vi "readRadonHtml.vi"(7 "Web(T)":bool=TRUE, 8 "Error In":errorcluster, 11 "url":string="http://localhost:80/radon.txt") -> (0 "Error Out":errorcluster, 1 "fechaMeas":string="17:44", 2 "fechaRead":string="25/05/1951", 3 "datoNuevo?":bool=TRUE, 4 "datosGraficaRadon":T1={"Radon"=0.0, "Temperature"=1100.0, "Humidity"=1050.25, "Pressure"=985.0, "Empty5"=885.75, "Empty6"=901.5, "Empty7"=970.5, "Empty8"=900.5} {"Empty8" format="%.1f"; "Empty7" format="%.1f"; "Empty6" format="%.1f"; "Empty5" format="%.1f"; "Pressure" format="%.1f"; "Humidity" format="%.1f"; "Temperature" format="%.1f"; "Radon" format="%.1f"})   [LabVIEW 2013]
uses:
  datosGraficaRadonNumeric.ctl
  <vilib>/httpClient/LabVIEWHTTPClient.lvlib
panel:
  out "body":string="1495730694 0,000000 1100,000000 1050,250000 985,000000 885,750000 901,500000 970,500000 900,500000 823,500000 1049,500000 913,250000 1013,250000 0,000000 927,500000 949,250000 1025,500000 1000,750000 905,500000 1050,250000 950,750000 0,250000 0,250000 0,000000 0,001000\r\n"
  out "headers":string="HTTP/1.1 200 OK\r\nDate: Wed, 31 May 2017 21:19:10 GMT\r\nServer: Apache/2.4.25 (Win32) OpenSSL/1.0.2j PHP/7.1.4\r\nLast-Modified: Tue, 30 May 2017 21:29:51 GMT\r\nETag: \"10f-550c480f7c17c\"\r\nAccept-Ranges: bytes\r\nContent-Length: 271\r\nContent-Type: text/plain\r\n\r\n"
  # "LEE EL FICHERO TXT ALMACENADO EN EL SERVIDOR WEB\nEXTRAE LOS VALORES ORDENADOS A UNA MATRIZ"
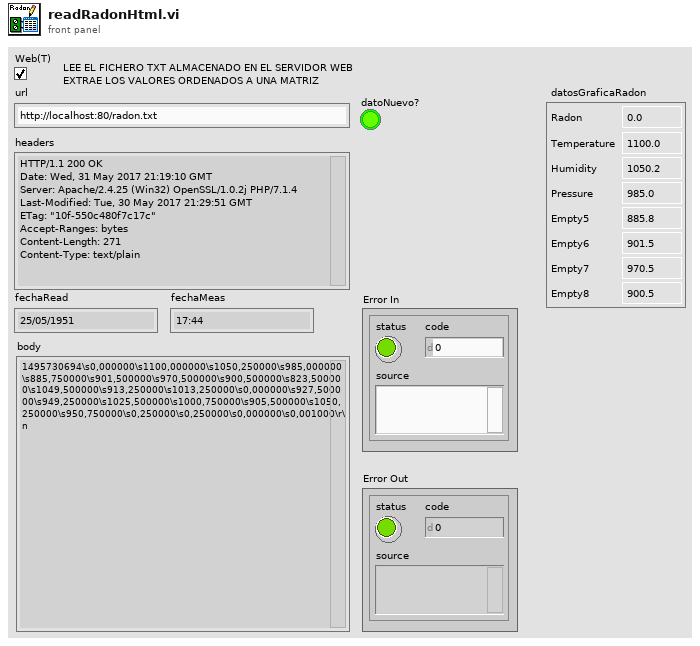
[diagram p1: front panel]
types:
  T1 = typedef "datosGraficaRadonNumeric.ctl" = cluster{"Radon":dbl, "Temperature":dbl, "Humidity":dbl, "Pressure":dbl, "Empty5":dbl, "Empty6":dbl, "Empty7":dbl, "Empty8":dbl}
  T2 = typedef "LabVIEWHTTPClient.lvlib/ClientHandle.ctl" = refnum<k1>
  T3 = cluster{"[0]":dbl, "[1]":dbl, "[2]":dbl, "[3]":dbl, "[4]":dbl, "[5]":dbl, "[6]":dbl, "[7]":dbl}
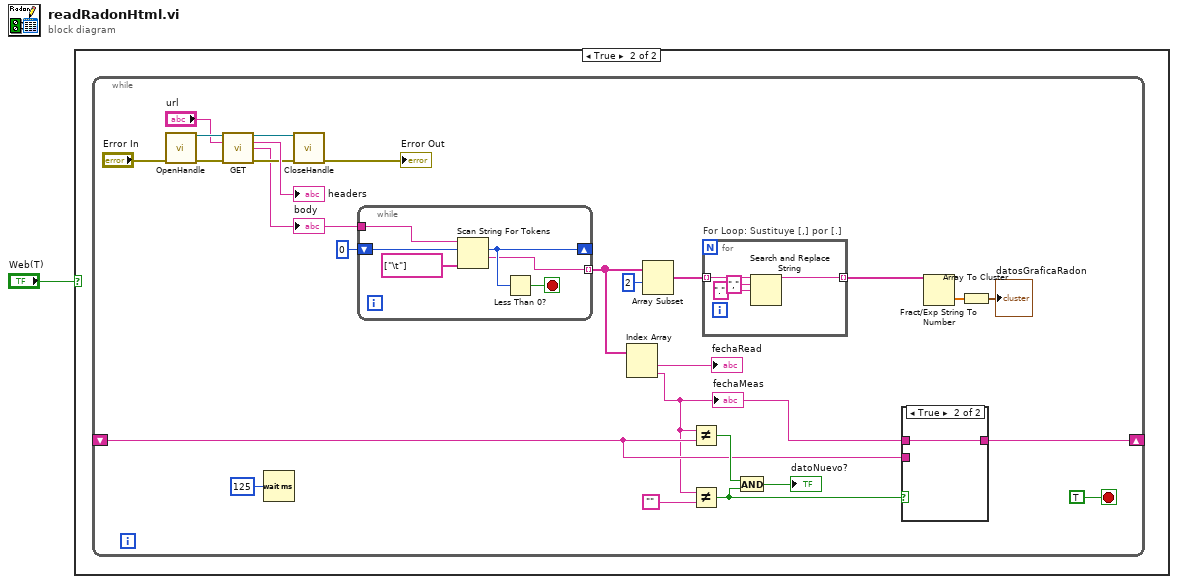
[diagram p0: block diagram]
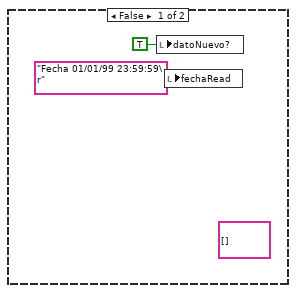
[diagram p2: hidden frame]
diagram:
  n1 = case shown="True" "Web(T)" {
    frame False {
      (unwired) string[][] []
      n2 = local write "datoNuevo?"(TRUE ("datoNuevo?")) -> ()
      n3 = local write "fechaRead"("Fecha 01/01/99 23:59:59\r" ("Fecha")) -> ()
    }
    frame True {
      n4 = while {
        shift-right: [w12] -> _
        shift-left: _ -> [w11]
        stop <- TRUE stop-if-true
        n5 = call <vilib>:"OpenHandle.vi"("error in (no error)"="Error In") -> ("client handle out"=w29:T2, "error out"=w25:errorcluster)  [unwired: 13 in]
        n6 = call <vilib>:"GET.vi"("client handle"=w29, "url"="url", "error in (no error)"=w25) -> ("client handle out"=w28:T2, "headers"=→"headers":string, "body"=w23:string, "error out"=w26:errorcluster)  [unwired: 9 in]
        "body" <- w23
        n7 = Wait (ms)(milliseconds to wait=u32 125) -> ()  [unwired: 1 out]
        n8 = call <vilib>:"CloseHandle.vi"("client handle"=w28, "error in (no error)"=w26) -> ("error out"=→"Error Out":errorcluster)  [unwired: 13 in]
        n9 = while {
          tunnel: w23 -> [w41]
          shift-right: [w37] -> _
          shift-left: 0 ("offset past token") -> [w39]
          tunnel: [w36] -> w18 mode=indexing
          stop <- w38 stop-if-true
          n10 = Scan String For Tokens(6:string[] ["\t"] ("delimiters (\\s,\\t,\\r,\\n)"), 8:w39, 9:w41) -> (1:w36:string, 2:w37:i32)  [unwired: 3 in, 2 out]
          n11 = Less Than 0?(x=w37) -> (x < 0?=w38:bool)
        }
        n12 = Index Array(array=w18) -> (element #1=→"fechaRead":string, element #2=w4:string)  [unwired: 2 in]
        "fechaMeas" <- w4
        n13 = Array Subset(array=w18, index=2) -> (w19:string[])  [unwired: 1 in]
        n14 = Not Equal?(x=w4, y=w11) -> (x != y?=w15:bool)
        n15 = Not Equal?(x=w4, y="") -> (x != y?=w13:bool)
        n16 = for "For Loop: Sustituye [,] por [.]" {
          tunnel: w19 -> [w35] mode=indexing
          tunnel: [w32] -> w6 mode=indexing
          n17 = Search and Replace String(input string=w35, search string=",", replace string="." ("replace string (\"\")")) -> (result string=w32:string)  [unwired: 5 in, 3 out]
        }
        n18 = And(x=w15, y=w13) -> (x .and. y?=→"datoNuevo?":bool)
        n19 = case shown="True" w13 {
          tunnel: w4 -> [_ w31]
          tunnel: [w30 w31] -> w12
          tunnel: w11 -> [w30 _]
          frame False {
          }
          frame True {
          }
        }
        n20 = Fract/Exp String To Number(string=w6) -> (number=w8:dbl[])  [unwired: 3 in, 1 out]
        n21 = Array To Cluster(array=w8) -> (cluster=→"datosGraficaRadon":T3)
      }
    }
  }
